vi "ma_sml_Last Stage FIR Filter Design.vi"(1 "oversampling rate":dbl=1.0 format="%.2f", 2 "alias protect in final transition":bool, 3 "stop band attenuation":enum16{"84 dB", "96 dB", "120 dB"}(ring)=enum."120 dB") -> (0 "h":dbl[](array[numeric]) format="%.2f")   [LabVIEW 2020, in "NI_MAPro.lvlib"]
uses:
  NI_MAPro.lvlib
  NI_AALBase.lvlib
panel:
  in  "debug?":bool
  out "Waveform Graph 2":dbl[](graph)
  out "ripple":dbl=0.00045449899249565306 format="%.2e"
  out "Waveform Graph":cluster{i32, dbl, dbl[]}(graph)
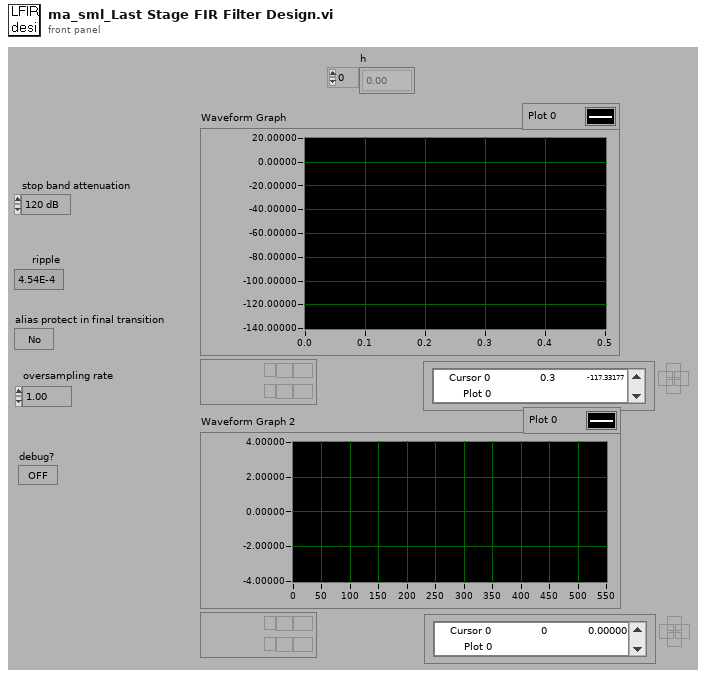
[diagram p1: front panel]
types:
  T1 = cluster{dbl, "oversampling rate":dbl, "oversampling rate":dbl, dbl}
  T2 = cluster{"Amplitude":dbl, "Lower Freq":dbl, "Higher Freq":dbl, "Weighted\nRipple":dbl}[]
  T3 = cluster{dbl, "oversampling rate":dbl, "oversampling rate":dbl, dbl}[]
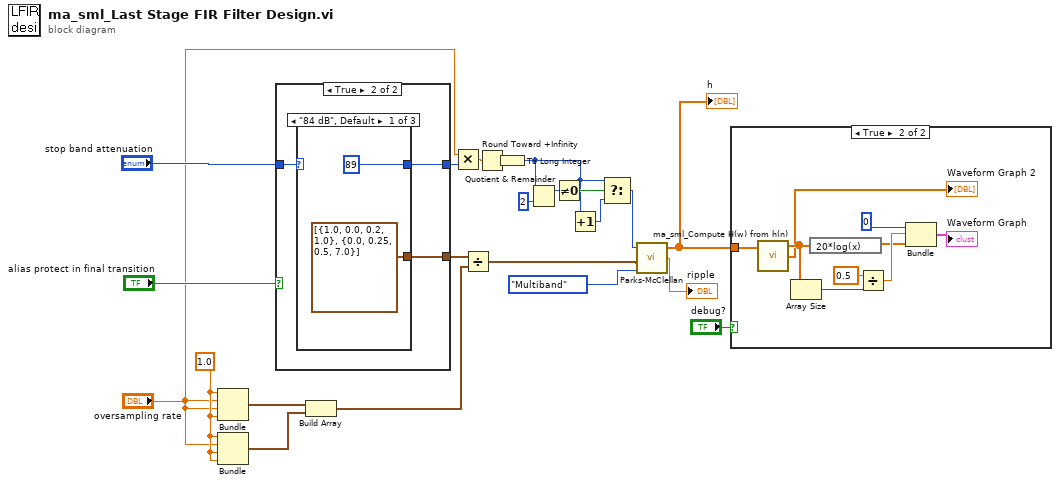
[diagram p0: block diagram]
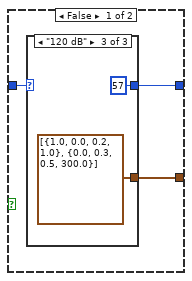
[diagram p3: hidden frame]
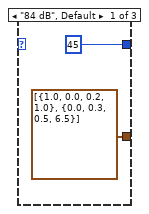
[diagram p4: hidden frame]
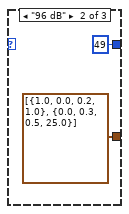
[diagram p5: hidden frame]
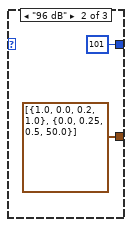
[diagram p6: hidden frame]
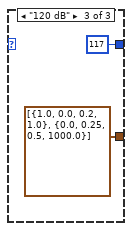
[diagram p7: hidden frame]
diagram:
  w16 = 1.0
  n1 = Bundle(w16, "oversampling rate"="oversampling rate", "oversampling rate"="oversampling rate", w16) -> (w17:T1)  [unwired: 1 out]
  n2 = Bundle(w16, "oversampling rate"="oversampling rate", w16, w16) -> (w15:cluster{dbl, "oversampling rate":dbl, dbl, dbl})  [unwired: 1 out]
  n3 = case shown="True" "alias protect in final transition" {
    tunnel: "stop band attenuation" -> [w25 w33]
    tunnel: [w24 w34] -> w10
    tunnel: [w23 w32] -> w14
    frame False {
      n4 = case shown="\"120 dB\"" w25 {
        tunnel: [45 49 57] -> w24
        tunnel: [T2 [{"Amplitude"=1.0, "Lower Freq"=0.0, "Higher Freq"=0.2, "Weighted\nRipple"=1.0}, {"Amplitude"=0.0, "Lower Freq"=0.3, "Higher Freq"=0.5, "Weighted\nRipple"=6.5}] ("Band Parameters") T2 [{"Amplitude"=1.0, "Lower Freq"=0.0, "Higher Freq"=0.2, "Weighted\nRipple"=1.0}, {"Amplitude"=0.0, "Lower Freq"=0.3, "Higher Freq"=0.5, "Weighted\nRipple"=25.0}] ("Band Parameters") T2 [{"Amplitude"=1.0, "Lower Freq"=0.0, "Higher Freq"=0.2, "Weighted\nRipple"=1.0}, {"Amplitude"=0.0, "Lower Freq"=0.3, "Higher Freq"=0.5, "Weighted\nRipple"=300.0}] ("Band Parameters")] -> w23
        frame "84 dB", Default {
        }
        frame "96 dB" {
        }
        frame "120 dB" {
        }
      }
    }
    frame True {
      n5 = case shown="\"84 dB\", Default" w33 {
        tunnel: [89 101 117] -> w34
        tunnel: [T2 [{"Amplitude"=1.0, "Lower Freq"=0.0, "Higher Freq"=0.2, "Weighted\nRipple"=1.0}, {"Amplitude"=0.0, "Lower Freq"=0.25, "Higher Freq"=0.5, "Weighted\nRipple"=7.0}] ("Band Parameters") T2 [{"Amplitude"=1.0, "Lower Freq"=0.0, "Higher Freq"=0.2, "Weighted\nRipple"=1.0}, {"Amplitude"=0.0, "Lower Freq"=0.25, "Higher Freq"=0.5, "Weighted\nRipple"=50.0}] ("Band Parameters") T2 [{"Amplitude"=1.0, "Lower Freq"=0.0, "Higher Freq"=0.2, "Weighted\nRipple"=1.0}, {"Amplitude"=0.0, "Lower Freq"=0.25, "Higher Freq"=0.5, "Weighted\nRipple"=1000.0}] ("Band Parameters")] -> w32
        frame "84 dB", Default {
        }
        frame "96 dB" {
        }
        frame "120 dB" {
        }
      }
    }
  }
  n6 = Build Array(w17, w15) -> (w13:T3)
  n7 = Multiply(x="oversampling rate", y=w10) -> (x*y=w11:dbl)
  n8 = Divide(x=w14, y=w13) -> (x/y=w12:cluster{dbl, dbl, dbl, dbl}[])
  n9 = Round Toward +Infinity(x=w11) -> (ceil(x): smallest int >= x=w8:dbl)
  n10 = To Long Integer(number=w8) -> (32bit integer=w3:i32)
  n11 = Quotient & Remainder(x=w3, y=2) -> (x-y*floor(x/y)=w6:i32)  [unwired: 1 out]
  n12 = Not Equal To 0?(x=w6) -> (x != 0?=w5:bool)
  n13 = Increment(x=w3) -> (x+1=w2:i32)
  n14 = Select(t=w3, s=w5, f=w2) -> (s? t:f=w4:i32)
  n15 = call "Parks-McClellan.vi"("filter type"=enum32{"Multiband", "Differentiator", "Hilbert"}."Multiband", "Band Parameters"=w12, "# of taps"=w4) -> ("ripple"=→"ripple":dbl, "h"=w18:dbl[])  [unwired: 1 in, 1 out]
  "h" <- w18
  n16 = case shown="True" "debug?" {
    tunnel: w18 -> [_ w43]
    frame False {
    }
    frame True {
      n17 = call "ma_sml_Compute H(w) from h(n).vi"("h"=w43) -> ("Mag H(w)"=w49:dbl[], "Phase H(w)"=→"Waveform Graph 2":dbl[])  [unwired: 1 in, 1 out]
      n18 = Array Size(array=w49) -> (size(s)=w47:i32)
      n19 = expression code="20*log(x)"(w49) -> (w41:dbl[])
      n20 = Divide(x=0.5, y=w47) -> (x/y=w46:dbl)
      n21 = Bundle(0, w46, "Mag H(w)"=w41) -> (→"Waveform Graph":cluster{i32, dbl, "Mag H(w)":dbl[]})  [unwired: 1 out]
    }
  }
